vi "SendMotorSpeedsLeedy.vi"(5 "B Speed":dbl, 6 "A Speed":dbl) -> (0 "B Speed Value":dbl, 1 "B Command":string, 2 "Characters Sent":dbl, 3 "A Speed Value":dbl, 4 "A Command":string)   [LabVIEW 2011]
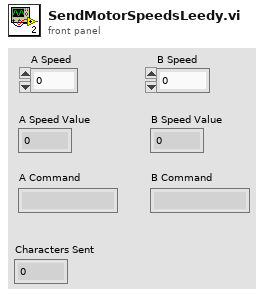
[diagram p1: front panel]
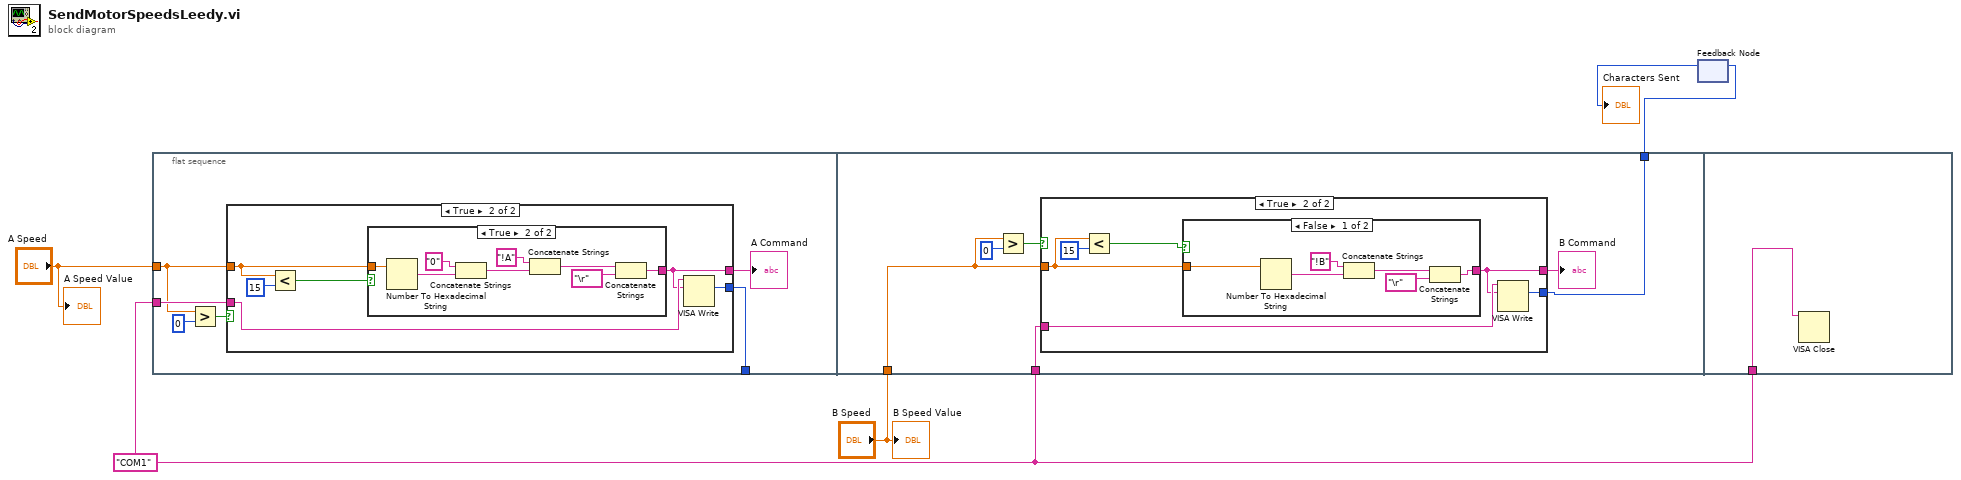
[diagram p0: block diagram]
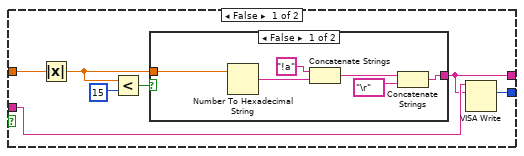
[diagram p2: hidden frame]
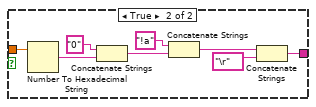
[diagram p3: hidden frame]
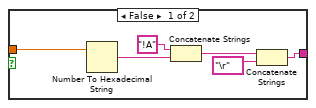
[diagram p4: hidden frame]
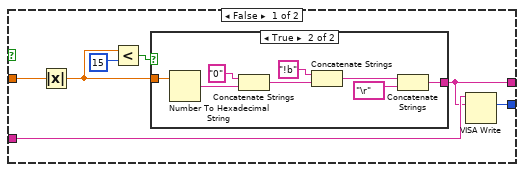
[diagram p5: hidden frame]
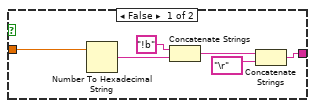
[diagram p6: hidden frame]
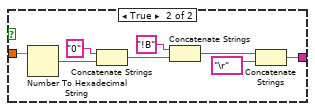
[diagram p7: hidden frame]
diagram:
  w1 = "COM1" ("Device Name")
  n1 = flat-sequence {
    tunnel: w1 -> [w10]
    tunnel: [w9] -> _
    tunnel: "A Speed" -> [w7]
    tunnel: "B Speed" -> [w56]
    tunnel: w1 -> [w55]
    tunnel: [w53] -> w2
    tunnel: w1 -> [w100]
    frame #0 {
      n2 = Greater?(x=w7, y=0) -> (0:w8:bool)
      n3 = case shown="True" w8 {
        tunnel: w7 -> [w18 w34]
        tunnel: w10 -> [w14 w37]
        tunnel: [w13 w36] -> w9
        tunnel: [w12 w35] -> w6
        frame False {
          n4 = Absolute Value(x=w18) -> (abs(x)=w15:dbl)
          n5 = Less?(x=w15, y=15) -> (x < y?=w16:bool)
          n6 = case shown="False" w16 {
            tunnel: w15 -> [w21 w26]
            tunnel: [w19 w25] -> w12
            frame False {
              n7 = Number To Hexadecimal String(2:w21) -> (0:w24:string)  [unwired: 1 in]
              n8 = Concatenate Strings("!a", w24) -> (w23:string)
              n9 = Concatenate Strings(w23, "\r") -> (w19:string)
            }
            frame True {
              n10 = Number To Hexadecimal String(2:w26) -> (0:w32:string)  [unwired: 1 in]
              n11 = Concatenate Strings("0", w32) -> (w30:string)
              n12 = Concatenate Strings("!a", w30) -> (w29:string)
              n13 = Concatenate Strings(w29, "\r") -> (w25:string)
            }
          }
          n14 = VISA Write(VISA resource name=w14, write buffer=w12) -> (return count=w13:u32)  [unwired: 1 in, 2 out]
        }
        frame True {
          n15 = Less?(x=w34, y=15) -> (x < y?=w33:bool)
          n16 = case shown="True" w33 {
            tunnel: w34 -> [w41 w46]
            tunnel: [w39 w45] -> w35
            frame False {
              n17 = Number To Hexadecimal String(2:w41) -> (0:w44:string)  [unwired: 1 in]
              n18 = Concatenate Strings("!A", w44) -> (w43:string)
              n19 = Concatenate Strings(w43, "\r") -> (w39:string)
            }
            frame True {
              n20 = Number To Hexadecimal String(2:w46) -> (0:w52:string)  [unwired: 1 in]
              n21 = Concatenate Strings("0", w52) -> (w50:string)
              n22 = Concatenate Strings("!A", w50) -> (w49:string)
              n23 = Concatenate Strings(w49, "\r") -> (w45:string)
            }
          }
          n24 = VISA Write(VISA resource name=w37, write buffer=w35) -> (return count=w36:u32)  [unwired: 1 in, 2 out]
        }
      }
      "A Command" <- w6
    }
    frame #1 {
      n25 = Greater?(x=w56, y=0) -> (0:w58:bool)
      n26 = case shown="True" w58 {
        tunnel: w56 -> [w65 w83]
        tunnel: w55 -> [w61 w82]
        tunnel: [w60 w81] -> w53
        tunnel: [w59 w80] -> w54
        frame False {
          n27 = Absolute Value(x=w65) -> (abs(x)=w62:dbl)
          n28 = Less?(x=w62, y=15) -> (x < y?=w63:bool)
          n29 = case shown="True" w63 {
            tunnel: w62 -> [w68 w73]
            tunnel: [w66 w72] -> w59
            frame False {
              n30 = Number To Hexadecimal String(2:w68) -> (0:w71:string)  [unwired: 1 in]
              n31 = Concatenate Strings("!b", w71) -> (w70:string)
              n32 = Concatenate Strings(w70, "\r") -> (w66:string)
            }
            frame True {
              n33 = Number To Hexadecimal String(2:w73) -> (0:w79:string)  [unwired: 1 in]
              n34 = Concatenate Strings("0", w79) -> (w77:string)
              n35 = Concatenate Strings("!b", w77) -> (w76:string)
              n36 = Concatenate Strings(w76, "\r") -> (w72:string)
            }
          }
          n37 = VISA Write(VISA resource name=w61, write buffer=w59) -> (return count=w60:u32)  [unwired: 1 in, 2 out]
        }
        frame True {
          n38 = Less?(x=w83, y=15) -> (x < y?=w84:bool)
          n39 = case shown="False" w84 {
            tunnel: w83 -> [w88 w92]
            tunnel: [w86 w93] -> w80
            frame False {
              n40 = Number To Hexadecimal String(2:w88) -> (0:w91:string)  [unwired: 1 in]
              n41 = Concatenate Strings("!B", w91) -> (w90:string)
              n42 = Concatenate Strings(w90, "\r") -> (w86:string)
            }
            frame True {
              n43 = Number To Hexadecimal String(2:w92) -> (0:w99:string)  [unwired: 1 in]
              n44 = Concatenate Strings("0", w99) -> (w97:string)
              n45 = Concatenate Strings("!B", w97) -> (w96:string)
              n46 = Concatenate Strings(w96, "\r") -> (w93:string)
            }
          }
          n47 = VISA Write(VISA resource name=w82, write buffer=w80) -> (return count=w81:u32)  [unwired: 1 in, 2 out]
        }
      }
      "B Command" <- w54
    }
    frame #2 {
      n48 = VISA Close(VISA resource name=w100) -> ()  [unwired: 1 in, 1 out]
    }
  }
  n49 = feedback #1() -> (→"Characters Sent":u32)  [unwired: 1 in]
  n50 = feedback-in #1(w2) -> ()
  "A Speed Value" <- "A Speed"
  "B Speed Value" <- "B Speed"
